vi "Config Type Def to Generic Type Defs.vi"(11 "measurement configuration":T12={"digital channel list"="7821\\PCMo 8", "frame clock rate"=48000.0, "number of channels"=2, "channel length"=32, "bit depth"=24, "data justification"=enum."Left Justified", "endianness"=enum."MSB First", "bit clock edge sync"=enum."Falling", "frame sync edge for channel 0"=enum."Falling", "channel 0 offset"=1, "master clock channel list"="7821\\PCMo 0", "master clock rate"=12288000.0, "enable dither"=TRUE, "logic level"=enum."3.3 V", "output level start"=-1.0, "output level stop"=20.0, "output sweep number of steps"=20000, "output level units"=enum."dBFS", "output range (pk-pk)"=15.0, "load impedance"=4.0, "signal phase"=0.0, "acq sampling rate"=51200.0, "min measurement cycles"=20, "min measurement time (s)"=0.1, "min settling cycles"=0, "min settling time (s)"=0.0, "acq channel"="", "band start"=20.0, "band stop"=20000.0, "weighting filter"=enum."A-weighting", "highpass filter"=enum."DC", "lowpass filter"=enum."No filter", "SNR units"=enum."dB", "THD+N units"=enum."dB", "THD units"=enum."dB", "gain units"=enum."dB", "power measurement method"=enum."DMM", "power measurement resource"="", "power supply voltage"=1.0, "power supply current limit"=0.0, "sense resistor (Ohms)"=0.05} {"load impedance" format="%0.2f"; "master clock rate" format="%#_6pHz"; "frame clock rate" format="%#_6pHz"}) -> (3 "single tone settings":T1={"digital channel list"="7821\\PCMo 8", "frame clock rate"=48000.0, "number of channels"=2, "channel length"=32, "bit depth"=24, "data justification"=enum."Left Justified", "endianness"=enum."MSB First", "bit clock edge sync"=enum."Falling", "frame sync edge for channel 0"=enum."Falling", "channel 0 offset"=1, "master clock channel list"="7821\\PCMo 0", "master clock rate"=12288000.0, "enable dither"=TRUE, "logic level"=enum."3.3 V", "signal frequency"=1000.0, "output level"=-1.0, "output level units"=enum."dBFS", "output range (pk-pk)"=15.0, "load impedance"=4.0, "signal phase"=0.0, "acq sampling rate"=51200.0, "min measurement cycles"=20, "min measurement time (s)"=0.1, "min settling cycles"=0, "min settling time (s)"=0.0, "acq channel"="", "band start"=20.0, "band stop"=20000.0, "weighting filter"=enum."A-weighting", "highpass filter"=enum."DC", "lowpass filter"=enum."No filter", "SNR units"=enum."dB", "THD+N units"=enum."dB", "THD units"=enum."dB", "gain units"=enum."dB"} {"signal phase" format="%0.2f"; "master clock rate" format="%#_6pHz"; "frame clock rate" format="%#_6pHz"})   [LabVIEW 2021, in "Efficiency Sweep_Class D Amplifier.lvlib"]
uses:
  Efficiency Sweep_Class D Amplifier.lvlib
  Measurement Configuration.ctl
  shared/controls/digital audio protocol/data justification.ctl
  shared/controls/digital audio protocol/endianness.ctl
  shared/controls/digital audio protocol/digital edge.ctl
  shared/controls/digital audio protocol/logic level.ctl
  shared/controls/digital output level units.ctl
  shared/controls/weighting filter.ctl
  shared/controls/highpass filter.ctl
  shared/controls/lowpass filter.ctl
  shared/controls/units - snr.ctl
  shared/controls/units - ratio.ctl
  shared/controls/power measurement method.ctl
  shared/controls/single tone measurement settings (HW).ctl
  shared/controls/audio controls.lvlib
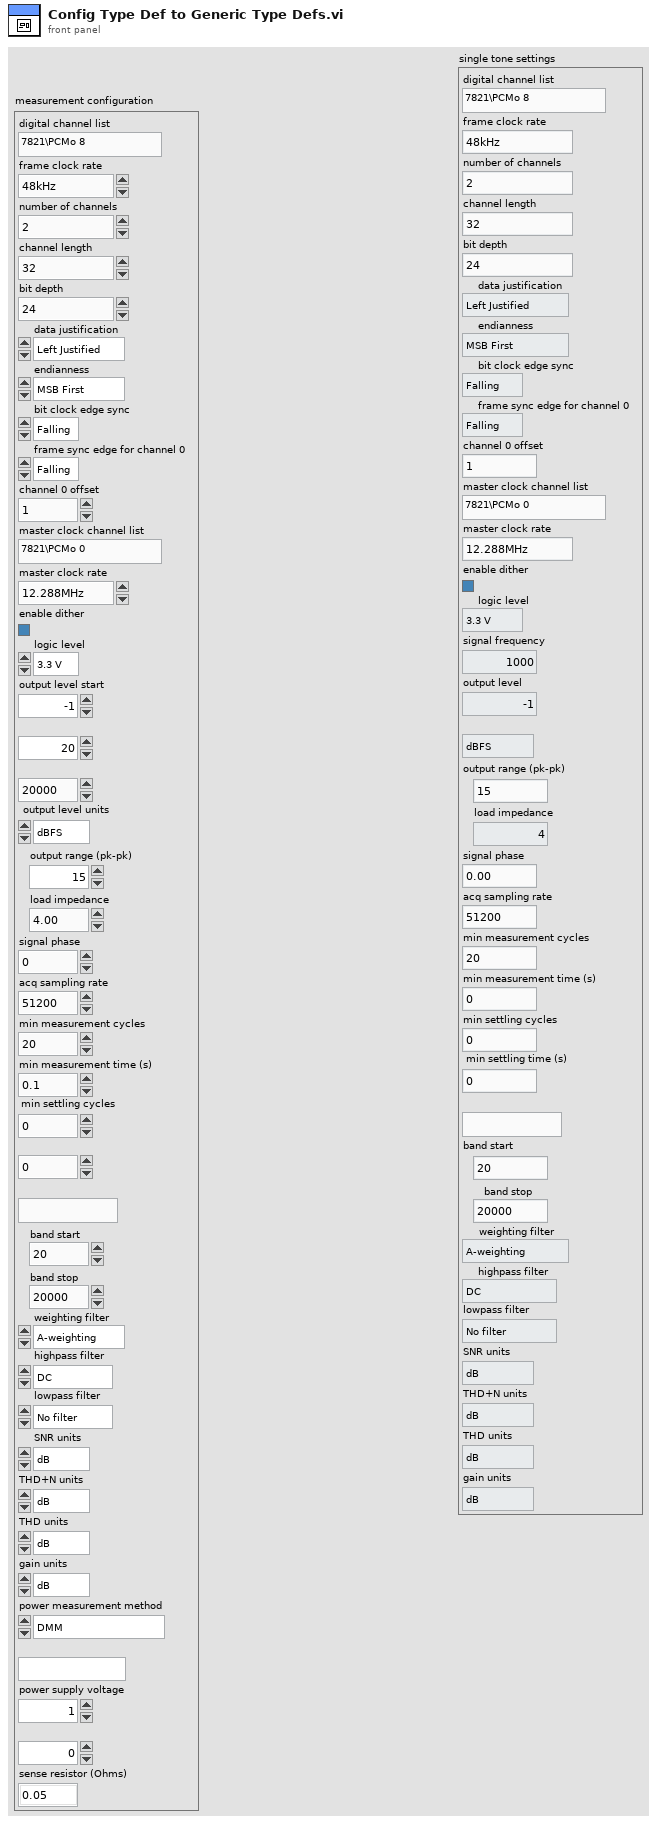
[diagram p1: front panel]
types:
  T1 = typedef "single tone measurement settings (HW).ctl" = cluster{"digital channel list":string, "frame clock rate":dbl, "number of channels":u32, "channel length":u32, "bit depth":u32, "data justification":T2, "endianness":T3, "bit clock edge sync":T4, "frame sync edge for channel 0":T4, "channel 0 offset":u32, "master clock channel list":string, "master clock rate":dbl, "enable dither":bool, "logic level":T5, "signal frequency":dbl, "output level":dbl, "output level units":T6, "output range (pk-pk)":dbl, "load impedance":dbl, "signal phase":dbl, "acq sampling rate":dbl, "min measurement cycles":u32, "min measurement time (s)":dbl, "min settling cycles":u32, "min settling time (s)":dbl, "acq channel":string, "band start":dbl, "band stop":dbl, "weighting filter":T7, "highpass filter":T8, "lowpass filter":T9, "SNR units":T10, "THD+N units":T11, "THD units":T11, "gain units":T11}
  T2 = typedef "data justification.ctl" = enum32{"Left Justified", "Right Justified"}
  T3 = typedef "endianness.ctl" = enum32{"MSB First", "LSB First"}
  T4 = typedef "digital edge.ctl" = enum32{"Rising", "Falling"}
  T5 = typedef "logic level.ctl" = enum32{"3.3 V", "1.8 V", "1.2 V"}
  T6 = typedef "audio controls.lvlib/digital output level units.ctl" = enum32{"% FS", "dBFS"}
  T7 = typedef "weighting filter.ctl" = enum32{"Linear", "A-weighting", "B-weighting", "C-weighting"}
  T8 = typedef "highpass filter.ctl" = enum32{"DC", "AC"}
  T9 = typedef "lowpass filter.ctl" = enum32{"No filter", "AES17 20kHz", "AES17 40kHz"}
  T10 = typedef "audio controls.lvlib/units - snr.ctl" = enum32{"dB", "x/y"}
  T11 = typedef "audio controls.lvlib/units - ratio.ctl" = enum32{"dB", "%", "x/y"}
  T12 = typedef "Efficiency Sweep_Class D Amplifier.lvlib/Measurement Configuration.ctl" = cluster{"digital channel list":string, "frame clock rate":dbl, "number of channels":u32, "channel length":u32, "bit depth":u32, "data justification":T2, "endianness":T3, "bit clock edge sync":T4, "frame sync edge for channel 0":T4, "channel 0 offset":u32, "master clock channel list":string, "master clock rate":dbl, "enable dither":bool, "logic level":T5, "output level start":dbl, "output level stop":dbl, "output sweep number of steps":u32, "output level units":T6, "output range (pk-pk)":dbl, "load impedance":dbl, "signal phase":dbl, "acq sampling rate":dbl, "min measurement cycles":u32, "min measurement time (s)":dbl, "min settling cycles":u32, "min settling time (s)":dbl, "acq channel":string, "band start":dbl, "band stop":dbl, "weighting filter":T7, "highpass filter":T8, "lowpass filter":T9, "SNR units":T10, "THD+N units":T11, "THD units":T11, "gain units":T11, "power measurement method":T13, "power measurement resource":string, "power supply voltage":dbl, "power supply current limit":dbl, "sense resistor (Ohms)":dbl}
  T13 = typedef "power measurement method.ctl" = enum32{"SMU", "DMM"}
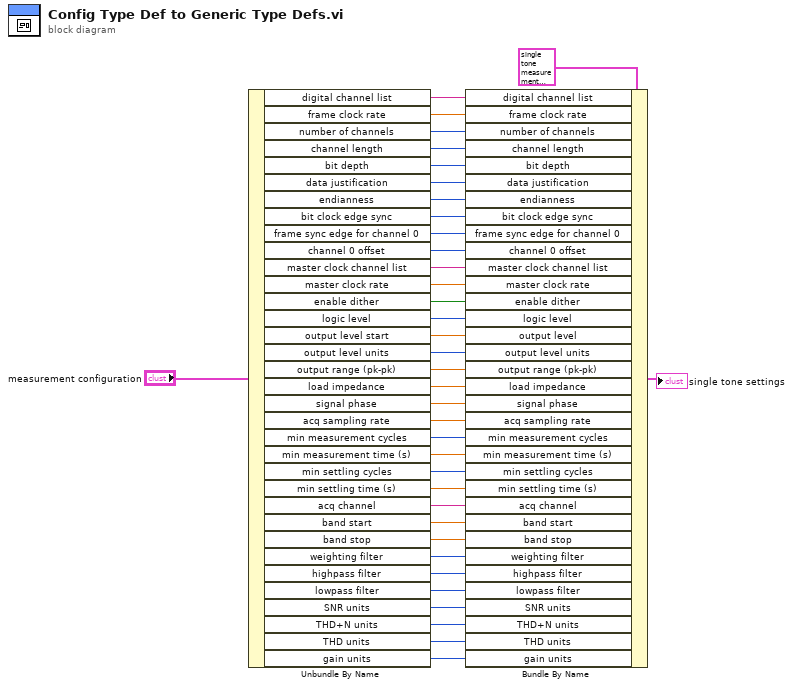
[diagram p0: block diagram]
diagram:
  n1 = Unbundle By Name("measurement configuration") -> ("digital channel list"=w34:string, "frame clock rate"=w33:dbl, "number of channels"=w32:u32, "channel length"=w31:u32, "bit depth"=w30:u32, "data justification"=w29:T2, "endianness"=w28:T3, "bit clock edge sync"=w27:T4, "frame sync edge for channel 0"=w26:T4, "channel 0 offset"=w25:u32, "master clock channel list"=w24:string, "master clock rate"=w23:dbl, "enable dither"=w22:bool, "logic level"=w21:T5, "output level start"=w1:dbl, "output level units"=w20:T6, "output range (pk-pk)"=w19:dbl, "load impedance"=w18:dbl, "signal phase"=w17:dbl, "acq sampling rate"=w16:dbl, "min measurement cycles"=w15:u32, "min measurement time (s)"=w14:dbl, "min settling cycles"=w13:u32, "min settling time (s)"=w12:dbl, "acq channel"=w11:string, "band start"=w10:dbl, "band stop"=w9:dbl, "weighting filter"=w8:T7, "highpass filter"=w7:T8, "lowpass filter"=w6:T9, "SNR units"=w5:T10, "THD+N units"=w4:T11, "THD units"=w3:T11, "gain units"=w2:T11)
  n2 = Bundle By Name(cluster=T1 {"digital channel list"="7821\\PCMo 8", "frame clock rate"=48000.0, "number of channels"=2, "channel length"=32, "bit depth"=24, "data justification"=enum."Left Justified", "endianness"=enum."MSB First", "bit clock edge sync"=enum."Falling", "frame sync edge for channel 0"=enum."Falling", "channel 0 offset"=1, "master clock channel list"="7821\\PCMo 0", "master clock rate"=12288000.0, "enable dither"=TRUE, "logic level"=enum."3.3 V", "signal frequency"=1000.0, "output level"=-1.0, "output level units"=enum."dBFS", "output range (pk-pk)"=15.0, "load impedance"=4.0, "signal phase"=0.0, "acq sampling rate"=51200.0, "min measurement cycles"=20, "min measurement time (s)"=0.1, "min settling cycles"=0, "min settling time (s)"=0.0, "acq channel"="", "band start"=20.0, "band stop"=20000.0, "weighting filter"=enum."A-weighting", "highpass filter"=enum."DC", "lowpass filter"=enum."No filter", "SNR units"=enum."dB", "THD+N units"=enum."dB", "THD units"=enum."dB", "gain units"=enum."dB"} ("measurement configuration"), "digital channel list"=w34, "frame clock rate"=w33, "number of channels"=w32, "channel length"=w31, "bit depth"=w30, "data justification"=w29, "endianness"=w28, "bit clock edge sync"=w27, "frame sync edge for channel 0"=w26, "channel 0 offset"=w25, "master clock channel list"=w24, "master clock rate"=w23, "enable dither"=w22, "logic level"=w21, "output level"=w1, "output level units"=w20, "output range (pk-pk)"=w19, "load impedance"=w18, "signal phase"=w17, "acq sampling rate"=w16, "min measurement cycles"=w15, "min measurement time (s)"=w14, "min settling cycles"=w13, "min settling time (s)"=w12, "acq channel"=w11, "band start"=w10, "band stop"=w9, "weighting filter"=w8, "highpass filter"=w7, "lowpass filter"=w6, "SNR units"=w5, "THD+N units"=w4, "THD units"=w3, "gain units"=w2) -> (→"single tone settings":T1)
